vi "TempScan.vi"() -> ()   [LabVIEW 2013]
panel:
  out "Last Completed Scan":cluster{dbl[], dbl[]}(graph)
  out "Temperature vs. Time":dbl(graph)=101.99
  out "Done?":bool=TRUE
  out "Time Remaining":dbl=-5.969752692180919e-10
  out "Power vs. Time":dbl(graph)=0.0004953086767793834
  out "Scan in progress":cluster{dbl[], dbl[]}(graph)
  in  "Delay Time between steps (s)":dbl=10.0 caption="Delay Time (s)"
  in  "Scan direction":bool
  in  "stop":bool
  in  "Step Size":dbl=0.01
  in  "High Temp":dbl=97.57
  in  "Low Temp":dbl=25.0
  out "Temp":dbl=101.99 format="%.2g"
  out "Setpoint":dbl=102.0 min=-99.0 max=250.0 step=0.01 format="%.2g"
  out "Voltage":dbl=-10.3 format="%.2g"
  out "Current":dbl=-3.02 format="%.2g"
  in  "TEC On":bool=TRUE
  in  "COM Port":u16=3
  # "Note: You may need to run the Arroyo Control\nprogram (Connect and then Exit) to wake up the\ntemperature controller and put it in remote mode."
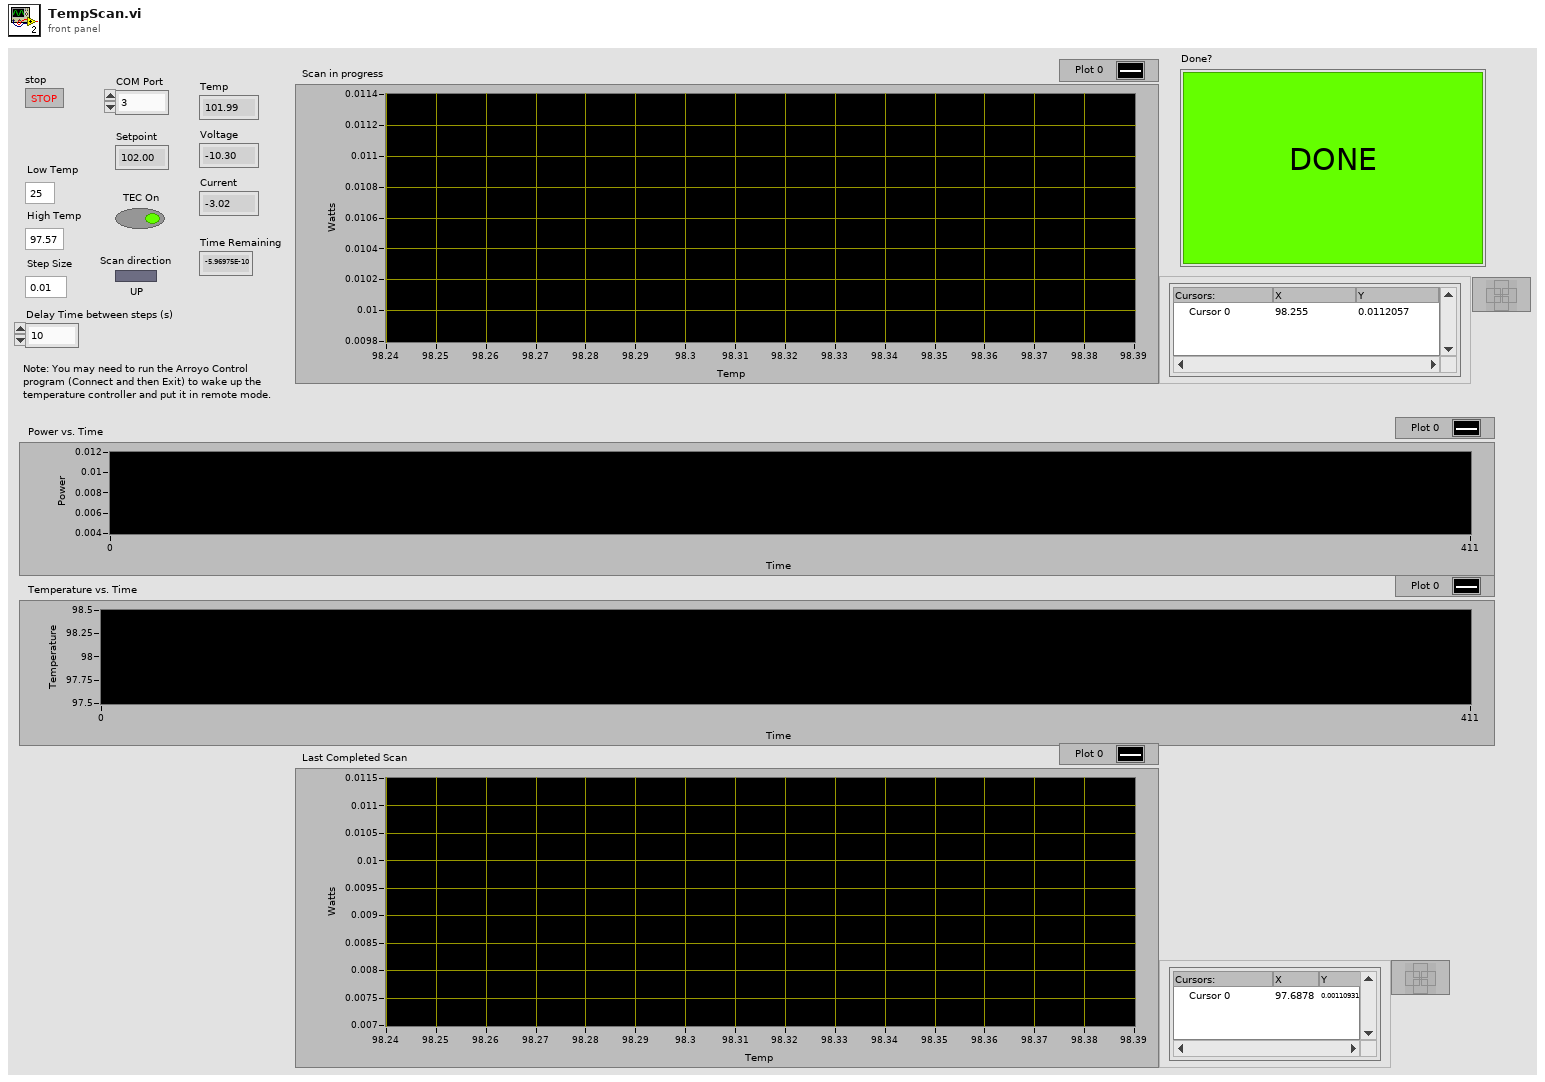
[diagram p1: front panel]
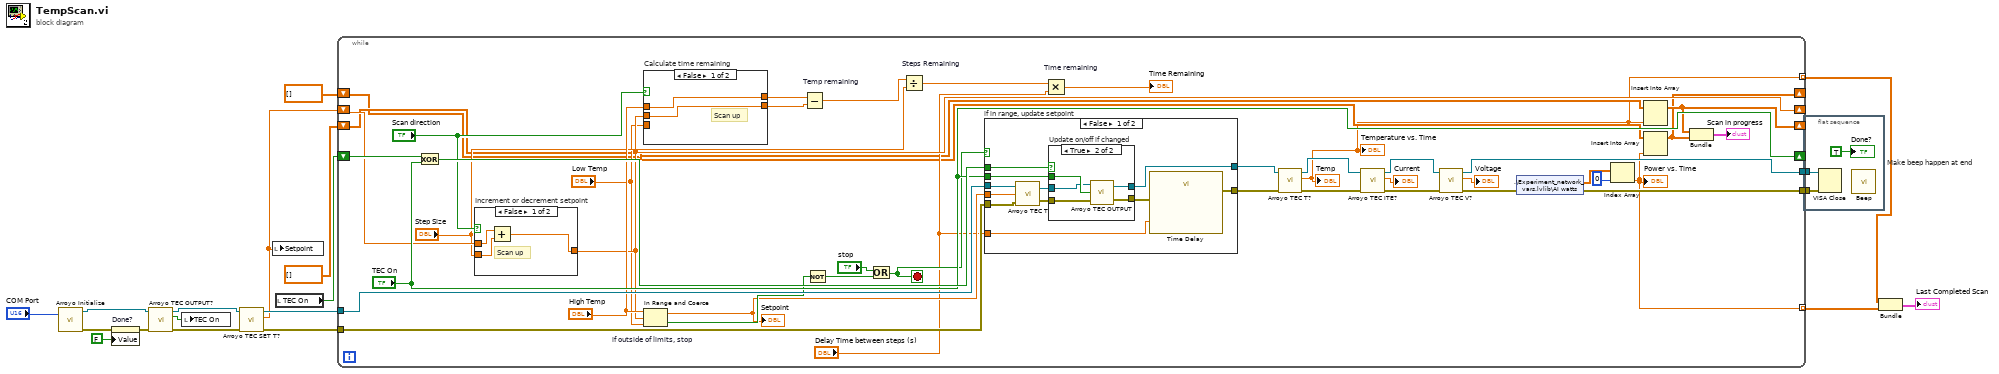
[diagram p0: block diagram]
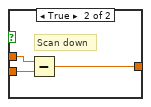
[diagram p5: hidden frame]
diagram:
  n1 = call "Arroyo Initialize.vi"("COM Port"="COM Port") -> ("dup VISA resource name"=w18:refnum<visa-resource-name>, "error out"=w7:errorcluster)  [unwired: 3 in]
  n2 = property on="Done?" class="Bool (strict)"(error in=w7, "Value"=FALSE ("Done?")) -> (error out=w6:errorcluster)  [unwired: 1 in, 1 out]
  n3 = call "Arroyo TEC OUTPUT?.vi"("error in (no error)"=w6, "VISA resource name"=w18) -> ("error out"=w16:errorcluster, "TEC Output"=w15:bool, "dup VISA resource name"=w17:refnum<visa-resource-name>)  [unwired: 3 in]
  n4 = local write "TEC On"(w15) -> ()
  n5 = call "Arroyo TEC SET T?.vi"("error in (no error)"=w16, "VISA resource name"=w17) -> ("error out"=w13:errorcluster, "TEC Temperature Setpoint"=w11:dbl, "dup VISA resource name"=w12:refnum<visa-resource-name>)  [unwired: 3 in]
  n6 = local write "Setpoint"(w11) -> ()
  n7 = local read "TEC On"() -> (w14:bool)
  n8 = while {
    tunnel: [w58] -> w9
    shift-right: ["TEC On"] -> _
    shift-left: w14 -> [w54]
    tunnel: w12 -> [w51]
    tunnel: w13 -> [w50]
    shift-right: [w37] -> _
    shift-left: w11 -> [w48]
    tunnel: [w28] -> w10
    shift-right: [w24] -> _
    shift-left: dbl[] [] -> [w26]
    shift-right: [w22] -> _
    shift-left: dbl[] [] -> [w23]
    tunnel: [w21] -> w2 mode=indexing
    tunnel: [w20] -> w1 mode=indexing
    stop <- w42 stop-if-true
    n9 = Exclusive Or(1:"TEC On", 2:w54) -> (0:w53:bool)
    n10 = case "Increment or decrement setpoint" shown="False" "Scan direction" {
      tunnel: "Step Size" -> [w88 w90]
      tunnel: [w86 w89] -> w37
      tunnel: w48 -> [w87 w91]
      frame False {
        # "Scan up"
        n11 = Add(x=w87, y=w88) -> (x+y=w86:dbl)
      }
      frame True {
        # "Scan down"
        n12 = Subtract(x=w91, y=w90) -> (x-y=w89:dbl)
      }
    }
    n13 = case "Calculate time remaining" shown="False" "Scan direction" {
      tunnel: "High Temp" -> [w63 _]
      tunnel: [w63 w65] -> w39
      tunnel: "Low Temp" -> [_ w64]
      tunnel: [w62 w64] -> w38
      tunnel: w37 -> [w62 w65]
      frame False {
        # "Scan up"
      }
      frame True {
        # "Scan down"
      }
    }
    n14 = In Range and Coerce "if outside of limits, stop"(upper limit="High Temp", x=w37, lower limit="Low Temp") -> (coerced(x)=w43:dbl, In Range?=w45:bool)
    "Setpoint" <- w43
    n15 = Subtract "Temp remaining"(x=w39, y=w38) -> (x-y=w36:dbl)
    n16 = Not(x=w45) -> (.not. x?=w44:bool)
    n17 = Or(x="stop", y=w44) -> (x .or. y?=w42:bool)
    n18 = Divide "Steps Remaining"(x=w36, y="Step Size") -> (x/y=w34:dbl)
    n19 = case "if in range, update setpoint" shown="False" w42 {
      tunnel: w53 -> [w76 _]
      tunnel: "TEC On" -> [w73 _]
      tunnel: w51 -> [w72 w84]
      tunnel: w50 -> [w71 w85]
      tunnel: [w70 w84] -> w49
      tunnel: [w68 w85] -> w46
      tunnel: w43 -> [w67 _]
      tunnel: "Delay Time between steps (s)" -> [w66 _]
      frame False {
        n20 = call "Arroyo TEC T.vi"("error in (no error)"=w71, "TEC Temperature Setpoint"=w67, "VISA resource name"=w72) -> ("error out"=w75:errorcluster, "dup VISA resource name"=w74:refnum<visa-resource-name>)
        n21 = case "Update on/off if changed" shown="True" w76 {
          tunnel: w73 -> [_ w83]
          tunnel: w75 -> [w77 w82]
          tunnel: w74 -> [w78 w81]
          tunnel: [w78 w80] -> w70
          tunnel: [w77 w79] -> w69
          frame False {
          }
          frame True {
            n22 = call "Arroyo TEC OUTPUT.vi"("error in (no error)"=w82, "TEC Output Enable"=w83, "VISA resource name"=w81) -> ("error out"=w79:errorcluster, "dup VISA resource name"=w80:refnum<visa-resource-name>)
          }
        }
        n23 = call "Time Delay"("error in (no error)"=w69, "Delay Time (s)"=w66) -> ("error out"=w68:errorcluster)  [unwired: 9 in]
      }
      frame True {
        # "stopping, don't update"
      }
    }
    n24 = Multiply "Time remaining"(x=w34, y="Delay Time between steps (s)") -> (x*y=→"Time Remaining":dbl)
    n25 = call "Arroyo TEC T?.vi"("error in (no error)"=w46, "VISA resource name"=w49) -> ("error out"=w59:errorcluster, "TEC Temperature"=w21:dbl, "dup VISA resource name"=w61:refnum<visa-resource-name>)  [unwired: 3 in]
    "Temp" <- w21
    "Temperature vs. Time" <- w21
    n26 = call "Arroyo TEC ITE?.vi"("error in (no error)"=w59, "VISA resource name"=w61) -> ("error out"=w57:errorcluster, "TEC Current"=→"Current":dbl, "dup VISA resource name"=w60:refnum<visa-resource-name>)  [unwired: 3 in]
    n27 = call "Arroyo TEC V?.vi"("error in (no error)"=w57, "VISA resource name"=w60) -> ("error out"=w29:errorcluster, "TEC Voltage"=→"Voltage":dbl, "dup VISA resource name"=w58:refnum<visa-resource-name>)  [unwired: 3 in]
    n28 = shared-variable ".\\Experiment_network_vars.lvlib\\AI watts"(error in=w29) -> (w30:dbl[], error out=w28:errorcluster)
    n29 = Index Array(array=w30, index=0) -> (element=w20:dbl)
    "Power vs. Time" <- w20
    n30 = Insert Into Array(array=w26, new element=w21) -> (w24:dbl[])  [unwired: 1 in]
    n31 = Insert Into Array(array=w23, new element=w20) -> (w22:dbl[])  [unwired: 1 in]
    n32 = Bundle(w24, w22) -> (→"Scan in progress":cluster{dbl[], dbl[]})  [unwired: 1 in]
  }
  n33 = flat-sequence "Make beep happen at end" {
    tunnel: w10 -> [w94]
    tunnel: w9 -> [w93]
    frame #0 {
      n34 = VISA Close(VISA resource name=w93, error in (no error)=w94) -> ()  [unwired: 1 out]
      n35 = call <vilib>:"Beep.vi"() -> ()  [unwired: 12 in]
      "Done?" <- TRUE ("Done?")
    }
  }
  n36 = Bundle(w2, w1) -> (→"Last Completed Scan":cluster{dbl[], dbl[]})  [unwired: 1 in]
